vi "UpdateSampleYupanInfo.vi"(0 "TCP网络连接输入":refnum<k5>, 1 "预判信息":string, 5 "Row":dbl, 7 "id":string, 9 "SampleTime":string, 11 "错误输入（无错误）":errorcluster) -> (6 "成功?":bool, 15 "错误输出":errorcluster)   [LabVIEW 2014]
panel:
  out "数据输出 2":string
  out "数据输出":string
  out "连接的字符串":string
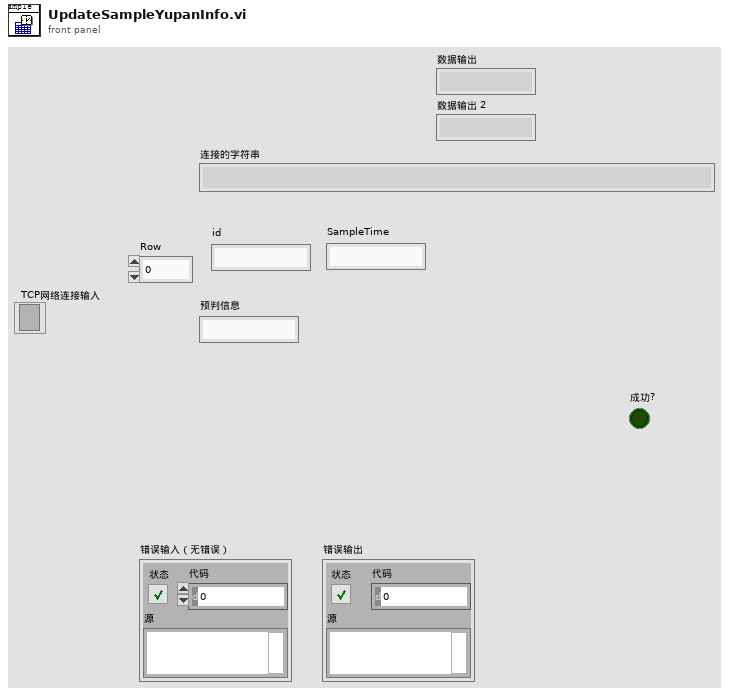
[diagram p1: front panel]
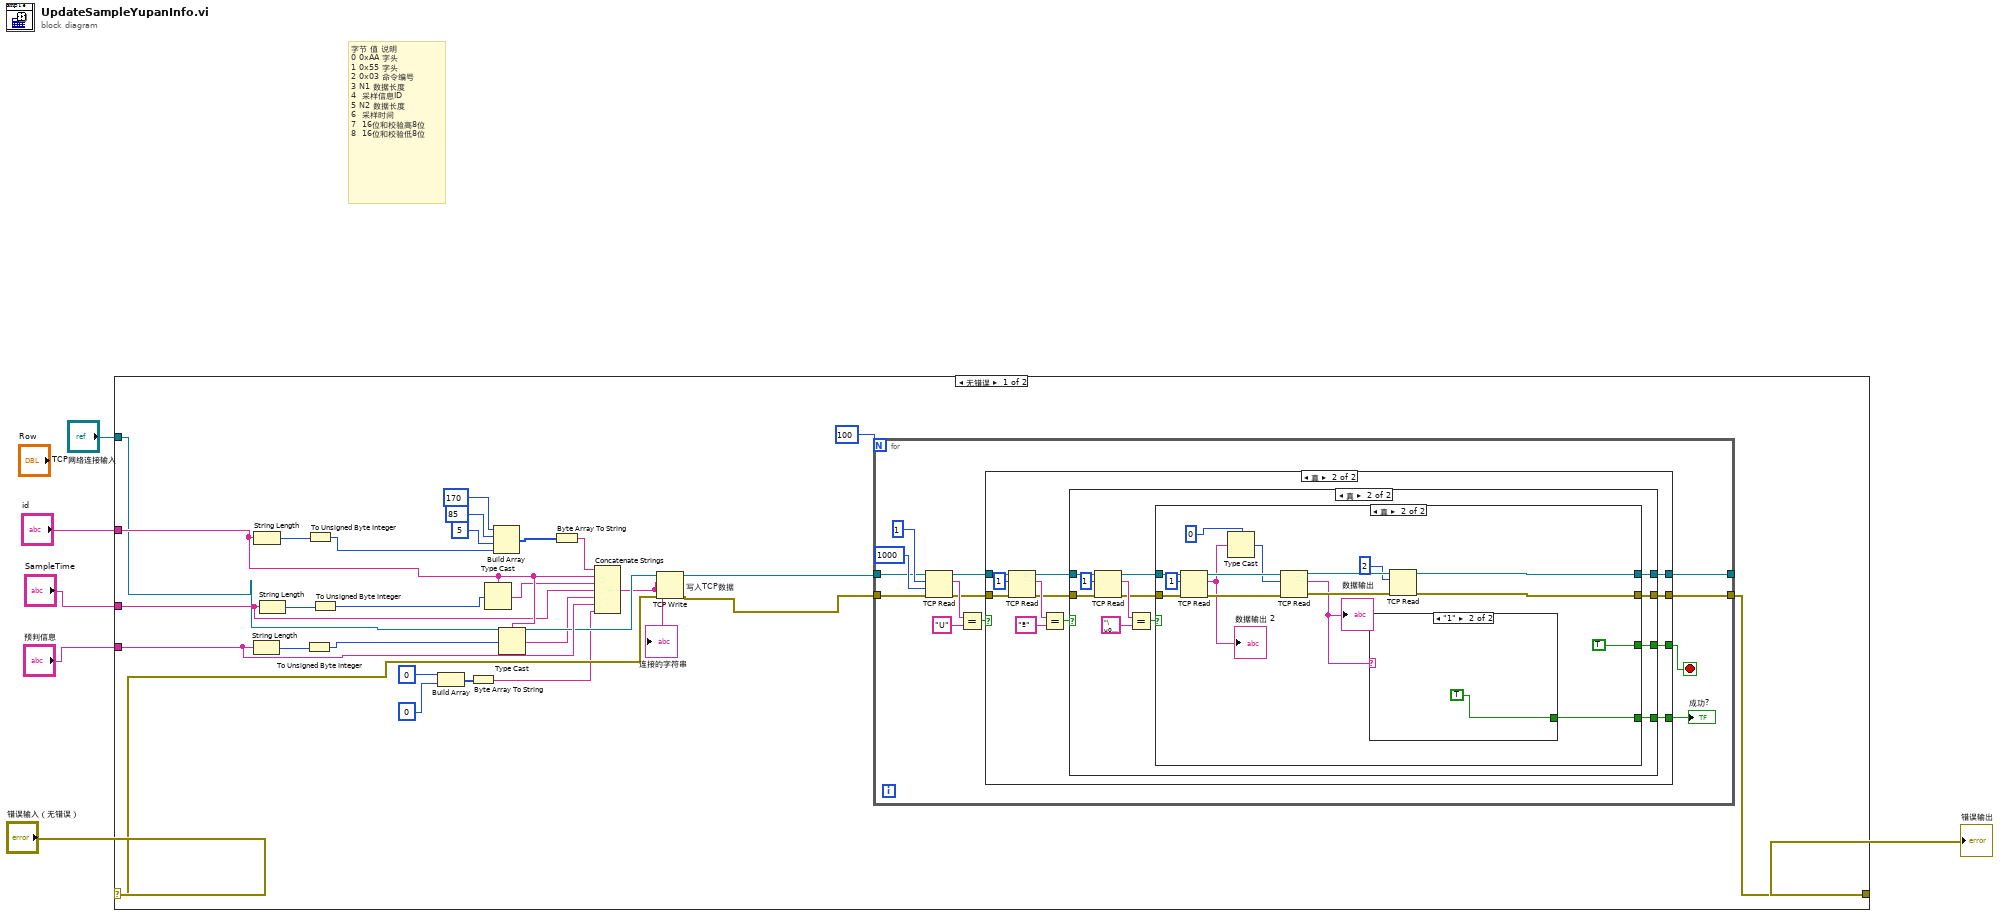
[diagram p0: block diagram]
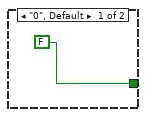
[diagram p5: hidden frame]
diagram:
  # "字节\t值\t说明\n0\t0xAA\t字头\n1\t0x55\t字头\n2\t0x03\t命令编号\n3\tN1\t数据长度\n4\t\t采样信息ID\n5\tN2\t数据长度\n6\t\t采样时间\n7\t\t16位和校验高8位\n8\t\t16位和校验低8位"
  n1 = case shown="无错误" "错误输入（无错误）" {
    selector: "错误输入（无错误）" -> [w23 w95]
    tunnel: [w22 w95] -> w6
    tunnel: "TCP网络连接输入" -> [w19 _]
    tunnel: "id" -> [w30 _]
    tunnel: "SampleTime" -> [w27 _]
    tunnel: "预判信息" -> [w24 _]
    frame No Error {
      n2 = String Length(string=w24) -> (length=w26:i32)
      n3 = String Length(string=w30) -> (length=w32:i32)
      n4 = String Length(string=w27) -> (length=w29:i32)
      n5 = To Unsigned Byte Integer(number=w26) -> (unsigned 8bit integer=w25:u8)
      n6 = To Unsigned Byte Integer(number=w32) -> (unsigned 8bit integer=w31:u8)
      n7 = To Unsigned Byte Integer(number=w29) -> (unsigned 8bit integer=w28:u8)
      n8 = Build Array(u8 0, u8 0) -> (w12:u8[])
      n9 = Byte Array To String(unsigned byte array=w12) -> (string=w7:string)
      n10 = Type Cast(type=w30, x=w28) -> (*(type *) &x=w9:string)
      n11 = Build Array(u8 170, u8 85, u8 5, w31) -> (w15:u8[])
      n12 = Type Cast(type=w30, x=w25) -> (*(type *) &x=w8:string)
      n13 = Byte Array To String(unsigned byte array=w15) -> (string=w11:string)
      n14 = Concatenate Strings(w11, w30, w9, w27, w8, w24, w7) -> (w10:string)
      "连接的字符串" <- w10
      n15 = TCP Write "写入TCP数据"(connection ID=w19, data in=w10, error in (no error)=w23) -> (connection ID out=w33:refnum<k5>, error out=w21:errorcluster)  [unwired: 1 in, 1 out]
      n16 = for "For循环" {
        N: 100 -> [_]
        tunnel: w33 -> [w39]
        tunnel: [w36] -> _
        tunnel: w21 -> [w38]
        tunnel: [w34] -> w22
        stop <- w37 stop-if-true
        n17 = TCP Read(connection ID=w39, bytes to read=1 ("读取的字节"), error in (no error)=w38, 9:1000 ("超时毫秒(25000)")) -> (connection ID out=w42:refnum<k5>, data out=w44:string, error out=w41:errorcluster)  [unwired: 1 in]
        n18 = Equal?(x=w44, y="U") -> (x = y?=w43:bool)
        n19 = case shown="真" w43 {
          tunnel: w42 -> [w48 w57]
          tunnel: w41 -> [w47 w56]
          tunnel: [w48 w52] -> w36
          tunnel: [w47 w51] -> w34
          tunnel: [_ w50] -> w37
          tunnel: [_ w49] -> w35
          frame False {
          }
          frame True {
            n20 = TCP Read(connection ID=w57, bytes to read=1 ("读取的字节"), error in (no error)=w56) -> (connection ID out=w54:refnum<k5>, data out=w58:string, error out=w53:errorcluster)  [unwired: 2 in]
            n21 = Equal?(x=w58, y="ª") -> (x = y?=w55:bool)
            n22 = case shown="真" w55 {
              tunnel: w54 -> [w62 w71]
              tunnel: w53 -> [w61 w70]
              tunnel: [w62 w66] -> w52
              tunnel: [w61 w65] -> w51
              tunnel: [_ w64] -> w50
              tunnel: [_ w63] -> w49
              frame False {
              }
              frame True {
                n23 = TCP Read(connection ID=w71, bytes to read=1 ("读取的字节"), error in (no error)=w70) -> (connection ID out=w69:refnum<k5>, data out=w72:string, error out=w68:errorcluster)  [unwired: 2 in]
                n24 = Equal?(x=w72, y="\u0005") -> (x = y?=w67:bool)
                n25 = case shown="真" w67 {
                  tunnel: w69 -> [w76 w91]
                  tunnel: w68 -> [w75 w90]
                  tunnel: [w76 w83] -> w66
                  tunnel: [w75 w84] -> w65
                  tunnel: [_ TRUE] -> w64
                  tunnel: [_ w77] -> w63
                  frame False {
                  }
                  frame True {
                    n26 = TCP Read(connection ID=w91, bytes to read=1 ("读取的字节"), error in (no error)=w90) -> (connection ID out=w89:refnum<k5>, data out=w81:string, error out=w88:errorcluster)  [unwired: 2 in]
                    "数据输出 2" <- w81
                    n27 = Type Cast(type=u8 0, x=w81) -> (*(type *) &x=w79:u8)
                    n28 = TCP Read(connection ID=w89, bytes to read=w79, error in (no error)=w88) -> (connection ID out=w86:refnum<k5>, data out=w78:string, error out=w85:errorcluster)  [unwired: 2 in]
                    "数据输出" <- w78
                    n29 = case shown="\"1\"" w78 {
                      tunnel: [FALSE TRUE] -> w77
                      frame "0", Default {
                      }
                      frame "1" {
                      }
                    }
                    n30 = TCP Read(connection ID=w86, bytes to read=2 ("读取的字节"), error in (no error)=w85) -> (connection ID out=w83:refnum<k5>, error out=w84:errorcluster)  [unwired: 2 in, 1 out]
                  }
                }
              }
            }
          }
        }
        "成功?" <- w35
      }
    }
    frame Error {
    }
  }
  "错误输出" <- w6
